vi "decrement N attempt.vi"(8 "error in (no error)":errorcluster, 11 "SP in":refnum<class "Save messages PGserver.lvclass">) -> (0 "error out":errorcluster, 2 "=0":bool, 3 "SP out":refnum<class "Save messages PGserver.lvclass">)   [LabVIEW 2019, in "Save messages PGserver.lvclass"]
uses:
  Save messages PGserver.lvclass
  Save messages PGserver.lvclass/Save messages PGserver.ctl
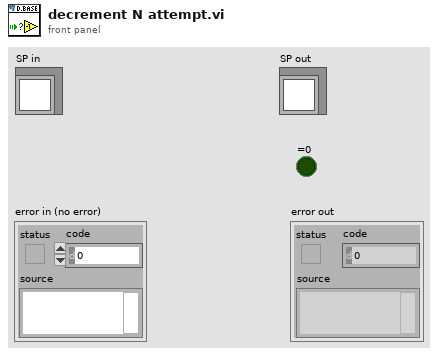
[diagram p1: front panel]
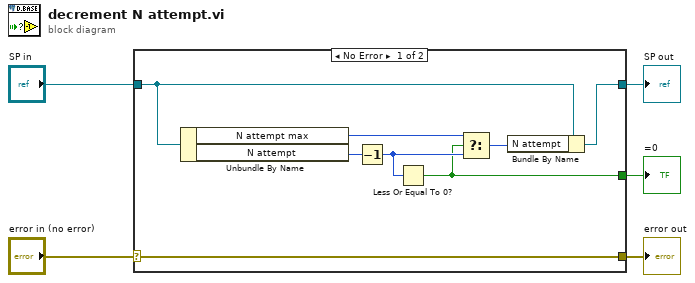
[diagram p0: block diagram]
diagram:
  n1 = case shown="No Error" "error in (no error)" {
    selector: "error in (no error)" -> [w13 w14]
    tunnel: [w13 w14] -> w4
    tunnel: [w12 w15] -> w1
    tunnel: "SP in" -> [w11 w15]
    tunnel: [w7 _] -> w3
    frame No Error {
      n2 = Unbundle By Name(w11) -> ("N attempt max"=w6:i32, "N attempt"=w10:i32)
      n3 = Decrement(x=w10) -> (x-1=w9:i32)
      n4 = Less Or Equal To 0?(x=w9) -> (x <= 0?=w7:bool)
      n5 = Select(t=w6, s=w7, f=w9) -> (s? t:f=w8:i32)
      n6 = Bundle By Name(cluster=w11, "N attempt"=w8) -> (w12:refnum<class "Save messages PGserver.lvclass">)
    }
    frame Error {
    }
  }
  "error out" <- w4
  "=0" <- w3
  "SP out" <- w1
